vi "setUp.vi"(8 "error in (no error)":errorcluster, 11 "reference in":refnum<class "FPGA Addon Adding Channel Items.lvclass">) -> (0 "error out":errorcluster, 3 "reference out":refnum<class "FPGA Addon Adding Channel Items.lvclass">)   [LabVIEW 2019, in "FPGA Addon Adding Channel Items.lvclass"]
doc: "setUp runs prior to the test method during test execution. Use this method to initialize any object data required by your tests."
uses:
  FPGA Addon Adding Channel Items.lvclass
  C:/Program Files (x86)/National Instruments/LabVIEW 2019/vi.lib/addons/_JKI Toolkits/VI Tester/TestCase.llb/TestCase.lvclass
  FPGA Addon Adding Channel Items.lvclass/FPGA Addon Adding Channel Items.ctl
  <vilib>/addons/_JKI Toolkits/VI Tester/TestCase.llb/TestCase.lvclass
  FPGA Addon Test Class/FPGA Addon Test Class.lvclass
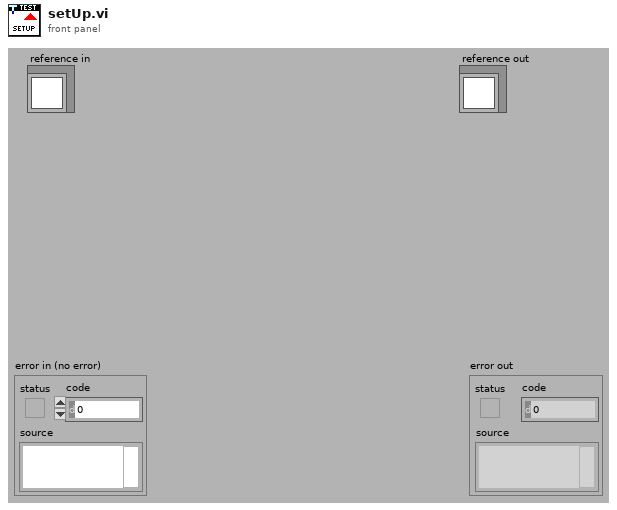
[diagram p1: front panel]
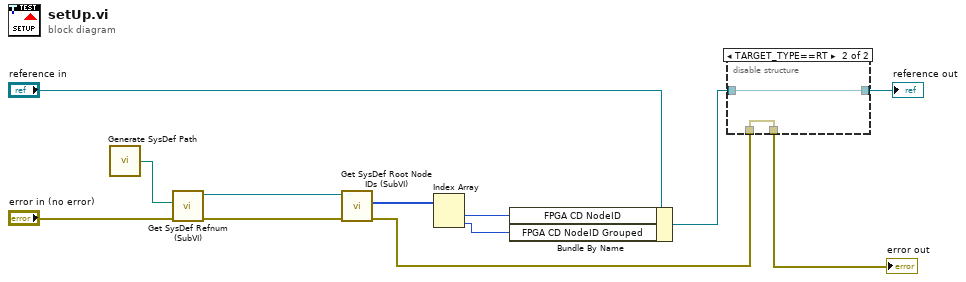
[diagram p0: block diagram]
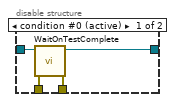
[diagram p2: hidden frame]
diagram:
  n1 = call "Generate SysDef Path.vi"() -> ("SysDef path"=w4:path)
  n2 = call "Get SysDef Refnum (SubVI).vi"("error in (no error)"="error in (no error)", "System Definition path"=w4) -> ("error out"=w8:errorcluster, "SysDef Refnum out"=w6:refnum<k24>)  [unwired: 8 in]
  n3 = call "Get SysDef Root Node IDs (SubVI).vi"("error in (no error)"=w8, "SysDef Refnum In"=w6) -> ("error out"=w7:errorcluster, "Root NodeIDs Out"=w3:u64[])  [unwired: 7 in, 1 out]
  n4 = Index Array(array=w3) -> (element #1=w2:u64, element #2=w1:u64)  [unwired: 2 in]
  n5 = Bundle By Name(cluster="reference in", "FPGA CD NodeID"=w2, "FPGA CD NodeID Grouped"=w1) -> (w9:refnum<class "FPGA Addon Adding Channel Items.lvclass">)
  n6 = disable-structure shown="TARGET_TYPE==RT" {
    disable-tunnel: w7 -> [w16 w17]
    disable-tunnel: [w15 w17] -> w12
    disable-tunnel: [w14 w18] -> w10
    disable-tunnel: w9 -> [w13 w18]
    frame condition #0 (active) {
      n7 = call <vilib>:"WaitOnTestComplete.vi"("error in (no error)"=w16, "TestCase in"=w13) -> ("error out"=w15:errorcluster, "TestCase out"=w14:refnum<class "FPGA Addon Adding Channel Items.lvclass">)  [unwired: 8 in]
    }
    frame condition #1 {
    }
  }
  "error out" <- w12
  "reference out" <- w10
